vi "H5Pset_fapl_multi.vi"(4 "Relax":bool, 6 "Member Address":u64, 7 "Member":i32(ring) items=["H5FD_MEM_NOLIST"=-1, "H5FD_MEM_DEFAULT"=0, "H5FD_MEM_SUPER"=1, "H5FD_MEM_BTREE"=2, "H5FD_MEM_DRAW"=3, "H5FD_MEM_GHEAP"=4, "H5FD_MEM_LHEAP"=5, "H5FD_MEM_OHDR"=6], 8 "error in (no error)":errorcluster, 9 "Member Name":string, 10 "Member FAPL":T1, 11 "HDF5 Property List Ref":T1) -> (0 "error out":errorcluster, 3 "HDF5 Property List Ref out":T1)   [LabVIEW 2017]
doc: "Sets up use of the multi-file driver."
uses:
  <vilib>/UPVI/lvhdf5/library.llb/HDF5 Ref.ctl
  <vilib>/UPVI/lvhdf5/hdf5.dll
panel:
  # "LVHDF5 Toolkit\nCopyright (c) 2005-2013 by Jason D. Sommerville\nCopyright (c) 2014 by UPVI, LLC.\n\nThis use and distribution of this file is governed by the terms found in \nLICENSE.txt distributed with this toolkit and installed at\n <user.lib>\\_lvhdf5\\LICENSE.txt"
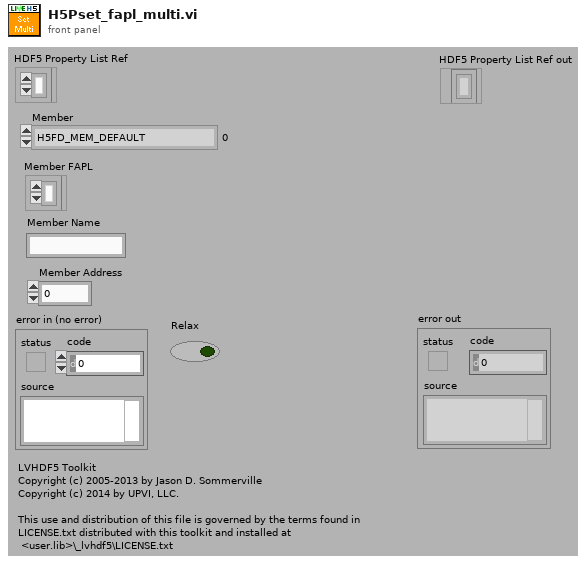
[diagram p1: front panel]
types:
  T1 = typedef "HDF5 Ref.ctl" = refnum<k1>
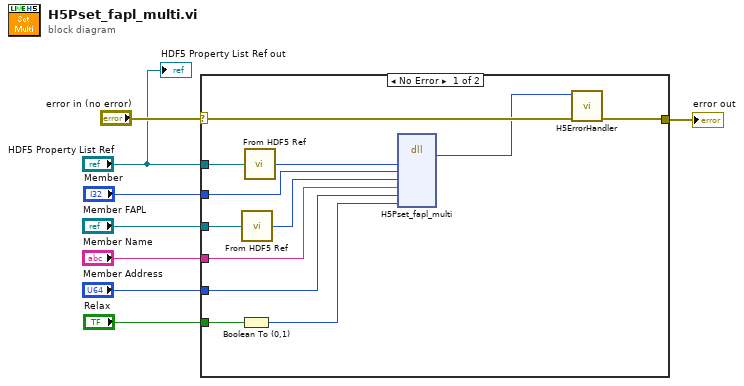
[diagram p0: block diagram]
diagram:
  n1 = case shown="No Error" "error in (no error)" {
    selector: "error in (no error)" -> [w20 w21]
    tunnel: [w19 w21] -> w7
    tunnel: "HDF5 Property List Ref" -> [w18 _]
    tunnel: "Member" -> [w15 _]
    tunnel: "Member FAPL" -> [w14 _]
    tunnel: "Member Name" -> [w12 _]
    tunnel: "Member Address" -> [w9 _]
    tunnel: "Relax" -> [w11 _]
    frame No Error {
      n2 = Boolean To (0,1)(Boolean=w11) -> (0, 1=w10:i16)
      n3 = call <vilib>:"From HDF5 Ref.vi"("HDF5 Ref"=w14) -> ("I32"=w13:i32)
      n4 = call <vilib>:"From HDF5 Ref.vi"("HDF5 Ref"=w18) -> ("I32"=w17:i32)
      n5 = dll-call lib="C:/Program Files/National Instruments/LabVIEW 2017/vi.lib/UPVI/lvhdf5/hdf5.dll" fn="H5Pset_fapl_multi"("plist_id"=w17, "memb_map"=w15, "memb_fapl"=w13, "memb_name"=w12, "memb_addr"=w9, "relax"=w10) -> ("return type"=w16:i32)  [unwired: 9 in, 2 out]
      n6 = call <vilib>:"H5ErrorHandler.vi"("error in (no error)"=w20, "herr_t"=w16) -> ("error out"=w19:errorcluster)  [unwired: 3 in, 4 out]
    }
    frame Error {
    }
  }
  "error out" <- w7
  "HDF5 Property List Ref out" <- "HDF5 Property List Ref"
